vi "Write Current Message.vi"(8 "error in (no error)":errorcluster, 10 "Current Msgs":string[](array[string]), 11 "System Log in":refnum<class "System Log.lvclass">) -> (0 "error out":errorcluster, 3 "System Log out":refnum<class "System Log.lvclass">)   [LabVIEW 2016, in "System Log.lvclass"]
uses:
  System Log.lvclass
  System Log.lvclass/System Log.ctl
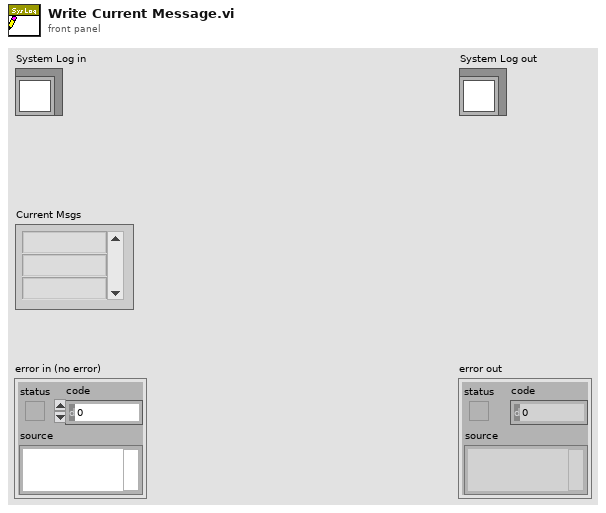
[diagram p1: front panel]
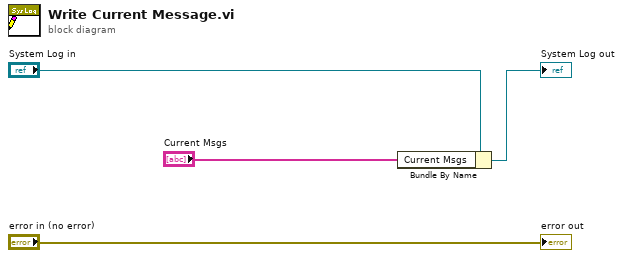
[diagram p0: block diagram]
diagram:
  n1 = Bundle By Name(cluster="System Log in", "Current Msgs"="Current Msgs") -> (→"System Log out":refnum<class "System Log.lvclass">)
  "error out" <- "error in (no error)"
